vi "Detect_peaks.vi"(9 "width":i32=3 min=3, 10 "Magnitude":waveform(dbl), 11 "Array":dbl[](array[numeric])) -> (2 "Locations":dbl[](array[numeric]), 3 "Peaks_xy":cluster{"Array":dbl[], "Amplitudes":dbl[]})   [LabVIEW 2015]
uses:
  <vilib>/Analysis/NI_AAL_SigProc.lvlib
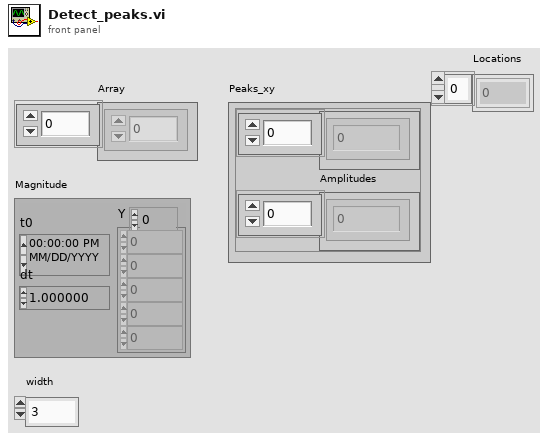
[diagram p1: front panel]
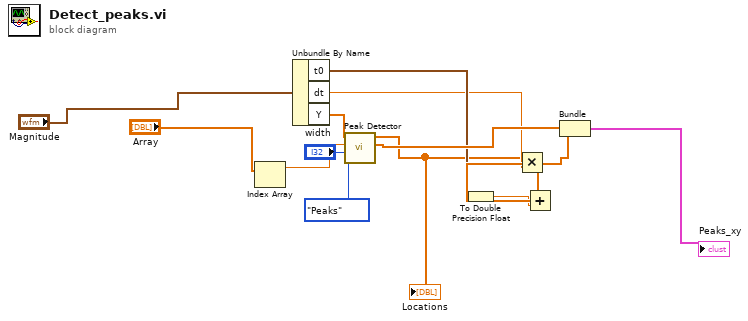
[diagram p0: block diagram]
diagram:
  n1 = Index Array(array="Array") -> (element=w2:dbl)  [unwired: 1 in]
  n2 = Unbundle By Name("Magnitude") -> ("t0"=w8:timestamp, "dt"=w6:dbl, "Y"=w3:dbl[])
  n3 = call <vilib>:"Peak Detector.vi"("peaks/valleys"=enum32{"Peaks", "Valleys"}."Peaks", "width"="width", "threshold"=w2, "X"=w3) -> ("Amplitudes"=w10:dbl[], "Locations"=w5:dbl[])  [unwired: 3 in, 3 out]
  "Locations" <- w5
  n4 = To Double Precision Float(number=w8) -> (double precision float=w9:dbl)
  n5 = Multiply(x=w5, y=w6) -> (x*y=w7:dbl[])
  n6 = Add(x=w7, y=w9) -> (x+y=w11:dbl[])
  n7 = Bundle(w11, "Amplitudes"=w10) -> (→"Peaks_xy":cluster{dbl[], "Amplitudes":dbl[]})  [unwired: 1 in]
